vi "Wave2D_Cal U_Apply BC_Y.vi"(8 "y length":i32, 9 "End Y Value":dbl[](array[numeric]), 10 "Start Y Value":dbl[](array[numeric]), 11 "U In":dbl[][](array[numeric])) -> (3 "U Out":dbl[][](array[numeric]))   [LabVIEW 2017, in "NI_PDE.lvlib"]
uses:
  <vilib>/gmath/NI_PDE.lvlib
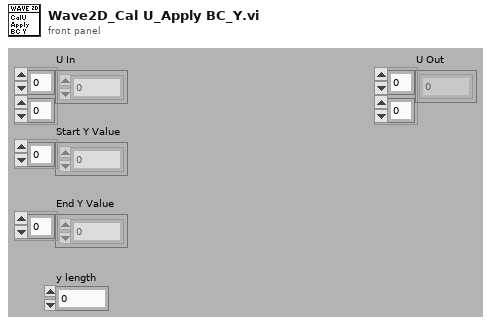
[diagram p1: front panel]
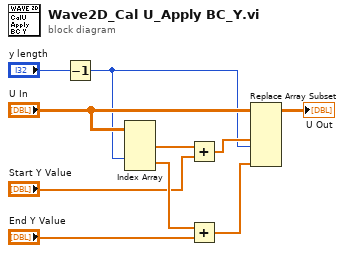
[diagram p0: block diagram]
diagram:
  n1 = Decrement(x="y length") -> (x-1=w4:i32)
  n2 = Index Array(array="U In", index (row) #2=w4) -> (element #1=w10:dbl[], element #2=w9:dbl[])  [unwired: 3 in]
  n3 = Add(x=w10, y="Start Y Value") -> (x+y=w8:dbl[])
  n4 = Add(x=w9, y="End Y Value") -> (x+y=w7:dbl[])
  n5 = Replace Array Subset(array="U In", new element #1=w8, new element #2=w7, index (row) #2=w4) -> (→"U Out":dbl[][])  [unwired: 3 in]
